vi "Non-Functioning.vi"() -> ()   [LabVIEW 2010]
doc: "This program dispalys a message to the user if the chosen mode of operation has not been programmed yet or is not operational for any reason."
panel:
  in  "OK Button":bool
  # "This Functionality Is Not\nYet Available.  Please \nTry Again Later."
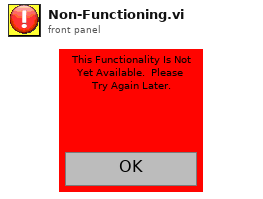
[diagram p1: front panel]
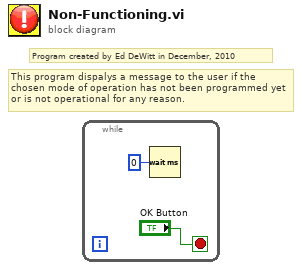
[diagram p0: block diagram]
diagram:
  # "This program dispalys a message to the user if the chosen mode of operation has not been programmed yet or is not operational for any reason."
  # "Program created by Ed DeWitt in December, 2010"
  n1 = while {
    stop <- "OK Button" stop-if-true
    n2 = Wait (ms)(milliseconds to wait=u32 0) -> ()  [unwired: 1 out]
  }
